vi "Initialization_K6221_ver1.0.vi"(4 "Input Comments String":string, 6 "output cluster":T1={"Main Sweep"=0, "Steps Config:"={"total points:"=0, "Step Delay (s)"=0.0, "Ini Delay (s)"=0.0, "# of steps:"=0}, "Temperature Control (ITC 503):"={"GPIB ADR"=0, "Change Heater?"={"Heater?"=FALSE, "Heater"=0}, "Change Temp?"={"Change T?"=FALSE, "Set T (K)"=0.0}, "Cluster"={"Heat Auto?"=FALSE, "Manual Heat?"=FALSE, "Heater (%)"=0.0}, "Change PID?"={"Change PID?"=FALSE, "P"=0.0, "I"=0.0, "D"=0.0}, "Change Para?"=FALSE, "Sensor"=1}, "Temperature Control (LS 340):"={"GPIB ADR"=0, "From (K)"=0.0, "To (K)"=0.0, "Rate (K/min)"=0.0, "Delta T (0.08K)"=0.0, "Temp. Header"="", "T Display Control"={"Ch B"=FALSE, "Ch C"=FALSE, "Ch D"=FALSE}}, "Magnet Control (IPS 120-10)"={"Action"=0, "Standby (s)"=0.0, "Heater on (s)"=0.0, "Sweep Setup "=[], "GPIB ADR"=0, "Change Para?"=FALSE}, "Keithley 6221 :"=[], "Measuring Instruments : "=[], "Lock-In SR7265 :"=[], "Deascription of \nthis measurement"="", "Instruments Config:"=[], "LS372 Bridge : 2"=[{"GPIB"=0, "Excitation"=0, "Autorange?"=FALSE, "Range"=0, "Current"=0, "Voltage"=0, "DataHeader"="Rx;Ry"}], "Magnet Control (CS4) 2"={"Action"=1, "Standby (s)"=0.0, "Heater on (s)"=300.0, "Sweep Setup "=[], "GPIB ADR"=0, "Change Para?"=FALSE}} {"Magnet Control (CS4) 2"."GPIB ADR" items=["None"=0, "25"=25]; "Magnet Control (CS4) 2"."Sweep Setup"."Rate in Range (T/min)" min=0.001 max=0.5 step=0.001; "Magnet Control (CS4) 2"."Sweep Setup"."Hold(min)" min=0.0; "Magnet Control (CS4) 2"."Sweep Setup"."Set Point (T)" min=-9.0 max=9.0 step=0.001; "Magnet Control (CS4) 2"."Action" items=["Up", "Down", "Pause", "Zero"]; "LS372 Bridge : 2"."Voltage" items=["2.00 uV"=1, "6.32 uV"=2, "20.0 uV"=3, "63.2 uV"=4, "200 uV"=5, "632 uV"=6, "2.0 mV"=7, "6.32 mV"=8]; "LS372 Bridge : 2"."Current" items=["1.00 pA"=1, "3.16 pA"=2, "10.0 pA"=3, "31.6 pA"=4, "100 pA"=5, "316 pA"=6, "1.00 nA"=7, "3.16 nA"=8, "10 nA"=9, "31.6 nA"=10, "100 nA"=11, "316 nA"=12, "1.00 uA"=13, "3.16 uA"=14, "10.0 uA"=15, "31.6 uA"=16, "100 uA"=17, "316 uA"=18, "1.00 mA"=19, "3.16 mA"=20, "10.0 mA"=21, "31.6 mA"=22]; "LS372 Bridge : 2"."Range" items=["2.0 m"=1, "6.32 m"=2, "20.0 m"=3, "63.2 m"=4, "200 m"=5, "632 m"=6, "2.00"=7, "6.32"=8, "20.0"=9, "63.2"=10, "200"=11, "632"=12, "2.00 k"=13, "6.32 k"=14, "20.0 k"=15, "63.2 k"=16, "200 k"=17, "632 k"=18, "2.00 M"=19, "6.32 M"=20, "20.0 M"=21, "63.2 M"=22]; "LS372 Bridge : 2"."Excitation" items=["Voltage", "Current"]; "LS372 Bridge : 2"."GPIB" items=["None"=0, "9"=9]; "Main Sweep" items=["Time", "DC Current", "Delta Current", "Pulse Delta Current", "Sine Current", "Lock-in Vosc"]; "Temperature Control (ITC 503):"."Sensor" items=["T2", "T3"]; "Magnet Control (IPS 120-10)"."Action" items=["Hold", "To Set point", "To Zero", "Clamp"]; "Keithley 6221 :"."Sweep Mode" items=["Linear", "Log", "Exp", "Inverse", "Manual"]}, 7 "error in (no error)":errorcluster, 10 "Input title array":string[](array[string])) -> (0 "error out":errorcluster, 1 "Output Comments string":string, 2 "output cluster 2":T1={"Main Sweep"=0, "Steps Config:"={"total points:"=0, "Step Delay (s)"=0.0, "Ini Delay (s)"=0.0, "# of steps:"=0}, "Temperature Control (ITC 503):"={"GPIB ADR"=0, "Change Heater?"={"Heater?"=FALSE, "Heater"=0}, "Change Temp?"={"Change T?"=FALSE, "Set T (K)"=0.0}, "Cluster"={"Heat Auto?"=FALSE, "Manual Heat?"=FALSE, "Heater (%)"=0.0}, "Change PID?"={"Change PID?"=FALSE, "P"=0.0, "I"=0.0, "D"=0.0}, "Change Para?"=FALSE, "Sensor"=1}, "Temperature Control (LS 340):"={"GPIB ADR"=0, "From (K)"=0.0, "To (K)"=0.0, "Rate (K/min)"=0.0, "Delta T (0.08K)"=0.0, "Temp. Header"="", "T Display Control"={"Ch B"=FALSE, "Ch C"=FALSE, "Ch D"=FALSE}}, "Magnet Control (IPS 120-10)"={"Action"=0, "Standby (s)"=0.0, "Heater on (s)"=0.0, "Sweep Setup "=[], "GPIB ADR"=0, "Change Para?"=FALSE}, "Keithley 6221 :"=[], "Measuring Instruments : "=[], "Lock-In SR7265 :"=[], "Deascription of \nthis measurement"="", "Instruments Config:"=[], "LS372 Bridge : 2"=[{"GPIB"=0, "Excitation"=0, "Autorange?"=FALSE, "Range"=0, "Current"=0, "Voltage"=0, "DataHeader"="Rx;Ry"}], "Magnet Control (CS4) 2"={"Action"=1, "Standby (s)"=0.0, "Heater on (s)"=300.0, "Sweep Setup "=[], "GPIB ADR"=0, "Change Para?"=FALSE}} {"Magnet Control (CS4) 2"."GPIB ADR" items=["None"=0, "25"=25]; "Magnet Control (CS4) 2"."Sweep Setup"."Rate in Range (T/min)" min=0.001 max=0.5 step=0.001; "Magnet Control (CS4) 2"."Sweep Setup"."Hold(min)" min=0.0; "Magnet Control (CS4) 2"."Sweep Setup"."Set Point (T)" min=-9.0 max=9.0 step=0.001; "Magnet Control (CS4) 2"."Action" items=["Up", "Down", "Pause", "Zero"]; "LS372 Bridge : 2"."Voltage" items=["2.00 uV"=1, "6.32 uV"=2, "20.0 uV"=3, "63.2 uV"=4, "200 uV"=5, "632 uV"=6, "2.0 mV"=7, "6.32 mV"=8]; "LS372 Bridge : 2"."Current" items=["1.00 pA"=1, "3.16 pA"=2, "10.0 pA"=3, "31.6 pA"=4, "100 pA"=5, "316 pA"=6, "1.00 nA"=7, "3.16 nA"=8, "10 nA"=9, "31.6 nA"=10, "100 nA"=11, "316 nA"=12, "1.00 uA"=13, "3.16 uA"=14, "10.0 uA"=15, "31.6 uA"=16, "100 uA"=17, "316 uA"=18, "1.00 mA"=19, "3.16 mA"=20, "10.0 mA"=21, "31.6 mA"=22]; "LS372 Bridge : 2"."Range" items=["2.0 m"=1, "6.32 m"=2, "20.0 m"=3, "63.2 m"=4, "200 m"=5, "632 m"=6, "2.00"=7, "6.32"=8, "20.0"=9, "63.2"=10, "200"=11, "632"=12, "2.00 k"=13, "6.32 k"=14, "20.0 k"=15, "63.2 k"=16, "200 k"=17, "632 k"=18, "2.00 M"=19, "6.32 M"=20, "20.0 M"=21, "63.2 M"=22]; "LS372 Bridge : 2"."Excitation" items=["Voltage", "Current"]; "LS372 Bridge : 2"."GPIB" items=["None"=0, "9"=9]; "Main Sweep" items=["Time", "DC Current", "Delta Current", "Pulse Delta Current", "Sine Current", "Lock-in Vosc"]; "Temperature Control (ITC 503):"."Sensor" items=["T2", "T3"]; "Magnet Control (IPS 120-10)"."Action" items=["Hold", "To Set point", "To Zero", "Clamp"]; "Keithley 6221 :"."Sweep Mode" items=["Linear", "Log", "Exp", "Inverse", "Manual"]}, 3 "Output title array":string[](array[string]), 8 "Output Mode Array":i32[](array[numeric]), 9 "VISA Refnum Out Array":refnum<visa-resource-name>[](array[refnum]))   [LabVIEW 2012]
doc: "Title Array: including time stamp, Temp (if selected), DCV, DCI, Vx, and Vy\nInstr GPIB ADR Array: If the instr is not selected, the GPIB ADR is equal to 0"
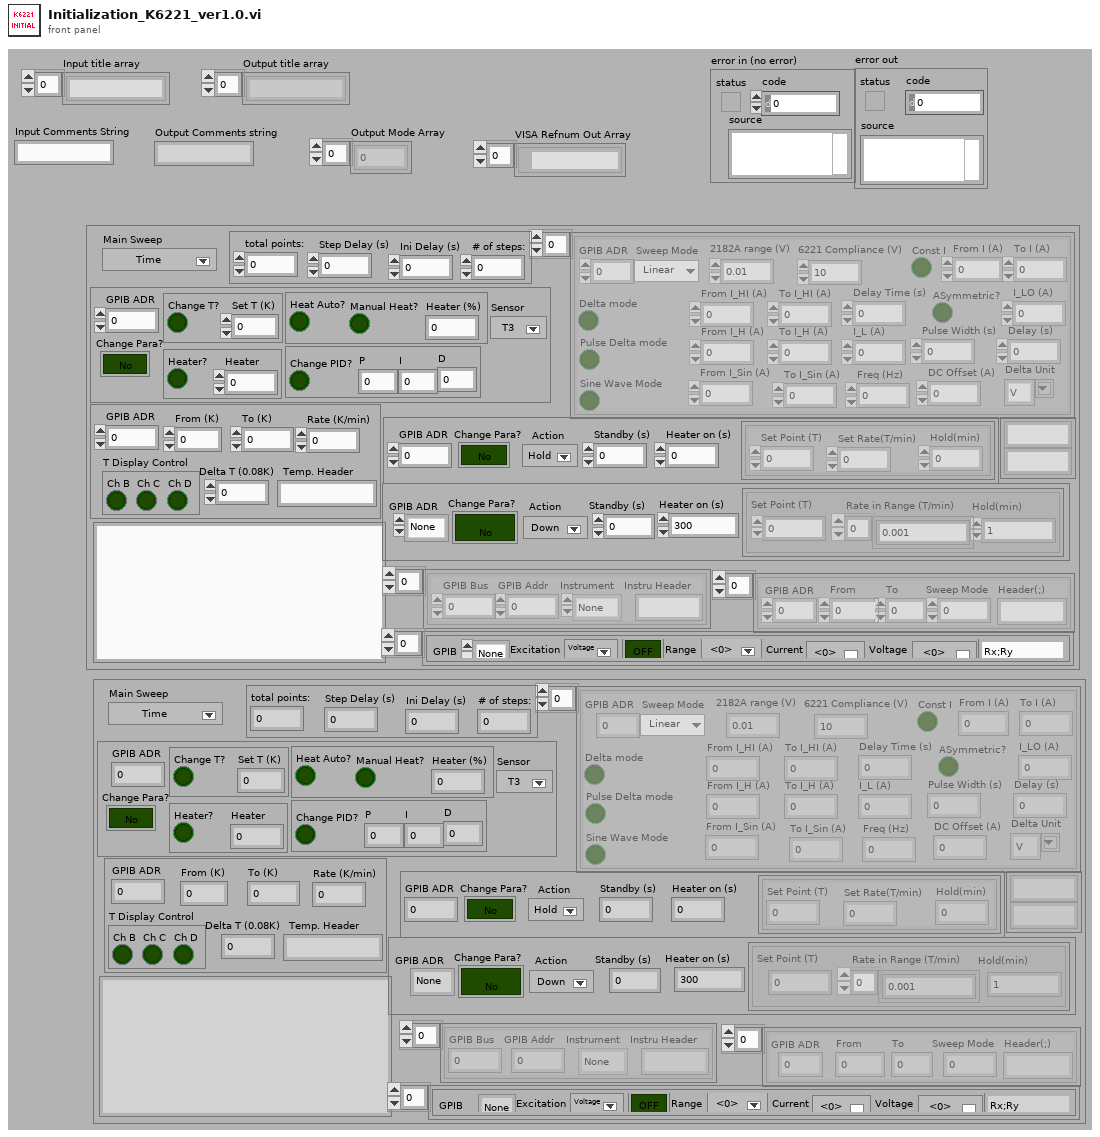
[diagram p1: front panel]
types:
  T1 = cluster{"Main Sweep":u8, "Steps Config:":cluster{"total points:":u32, "Step Delay (s)":dbl, "Ini Delay (s)":dbl, "# of steps:":u32}, "Temperature Control (ITC 503):":cluster{"GPIB ADR":u16, "Change Heater?":cluster{"Heater?":bool, "Heater":u8}, "Change Temp?":cluster{"Change T?":bool, "Set T (K)":dbl}, "Cluster":cluster{"Heat Auto?":bool, "Manual Heat?":bool, "Heater (%)":dbl}, "Change PID?":cluster{"Change PID?":bool, "P":dbl, "I":dbl, "D":dbl}, "Change Para?":bool, "Sensor":u16}, "Temperature Control (LS 340):":cluster{"GPIB ADR":u16, "From (K)":dbl, "To (K)":dbl, "Rate (K/min)":dbl, "Delta T (0.08K)":dbl, "Temp. Header":string, "T Display Control":cluster{"Ch B":bool, "Ch C":bool, "Ch D":bool}}, "Magnet Control (IPS 120-10)":cluster{"Action":u16, "Standby (s)":dbl, "Heater on (s)":dbl, "Sweep Setup ":cluster{"Set Point (T)":dbl, "Set Rate(T/min)":dbl, "Hold(min)":dbl}[], "GPIB ADR":u16, "Change Para?":bool}, "Keithley 6221 :":cluster{"Delta mode":bool, "Const I":bool, "Pulse Delta mode":bool, "Sine Wave Mode":bool, "From I_HI (A)":dbl, "From I (A)":dbl, "I_LO (A)":dbl, "From I_H (A)":dbl, "I_L (A)":dbl, "Freq (Hz)":dbl, "From I_Sin (A)":dbl, "DC Offset (A)":dbl, "Delay Time (s)":dbl, "Pulse Width (s)":dbl, "Delay (s)":dbl, "To I (A)":dbl, "ASymmetric?":bool, "To I_HI (A)":dbl, "To I_H (A)":dbl, "To I_Sin (A)":dbl, "GPIB ADR":u16, "Sweep Mode":u8, "Delta Unit":string, "2182A range (V)":dbl, "6221 Compliance (V)":dbl}[], "Measuring Instruments : ":cluster{"GPIB Bus":dbl, "GPIB Addr":dbl, "Instrument":enum16{"None", "HP34401DMM", "Lockin 7265", "HP3456/7A", "HP3478A", "HP3325FG", "Keithley2182A"}, "Instru Header":string}[], "Lock-In SR7265 :":cluster{"GPIB ADR":u16, "From":dbl, "To":dbl, "Header(;)":string, "Sweep Mode":u8}[], "Deascription of \nthis measurement":string, "Instruments Config:":string[][], "LS372 Bridge : 2":cluster{"GPIB":u16, "Excitation":u16, "Autorange?":bool, "Range":u16, "Current":u16, "Voltage":u16, "DataHeader":string}[], "Magnet Control (CS4) 2":cluster{"Action":u16, "Standby (s)":dbl, "Heater on (s)":dbl, "Sweep Setup ":cluster{"Set Point (T)":dbl, "Hold(min)":dbl, "Rate in Range (T/min)":dbl[]}[], "GPIB ADR":u16, "Change Para?":bool}}
  T2 = cluster{"Delta mode":bool, "Const I":bool, "Pulse Delta mode":bool, "Sine Wave Mode":bool, "From I_HI (A)":dbl, "From I (A)":dbl, "I_LO (A)":dbl, "From I_H (A)":dbl, "I_L (A)":dbl, "Freq (Hz)":dbl, "From I_Sin (A)":dbl, "DC Offset (A)":dbl, "Delay Time (s)":dbl, "Pulse Width (s)":dbl, "Delay (s)":dbl, "To I (A)":dbl, "ASymmetric?":bool, "To I_HI (A)":dbl, "To I_H (A)":dbl, "To I_Sin (A)":dbl, "GPIB ADR":u16, "Sweep Mode":u8, "Delta Unit":string, "2182A range (V)":dbl, "6221 Compliance (V)":dbl}[]
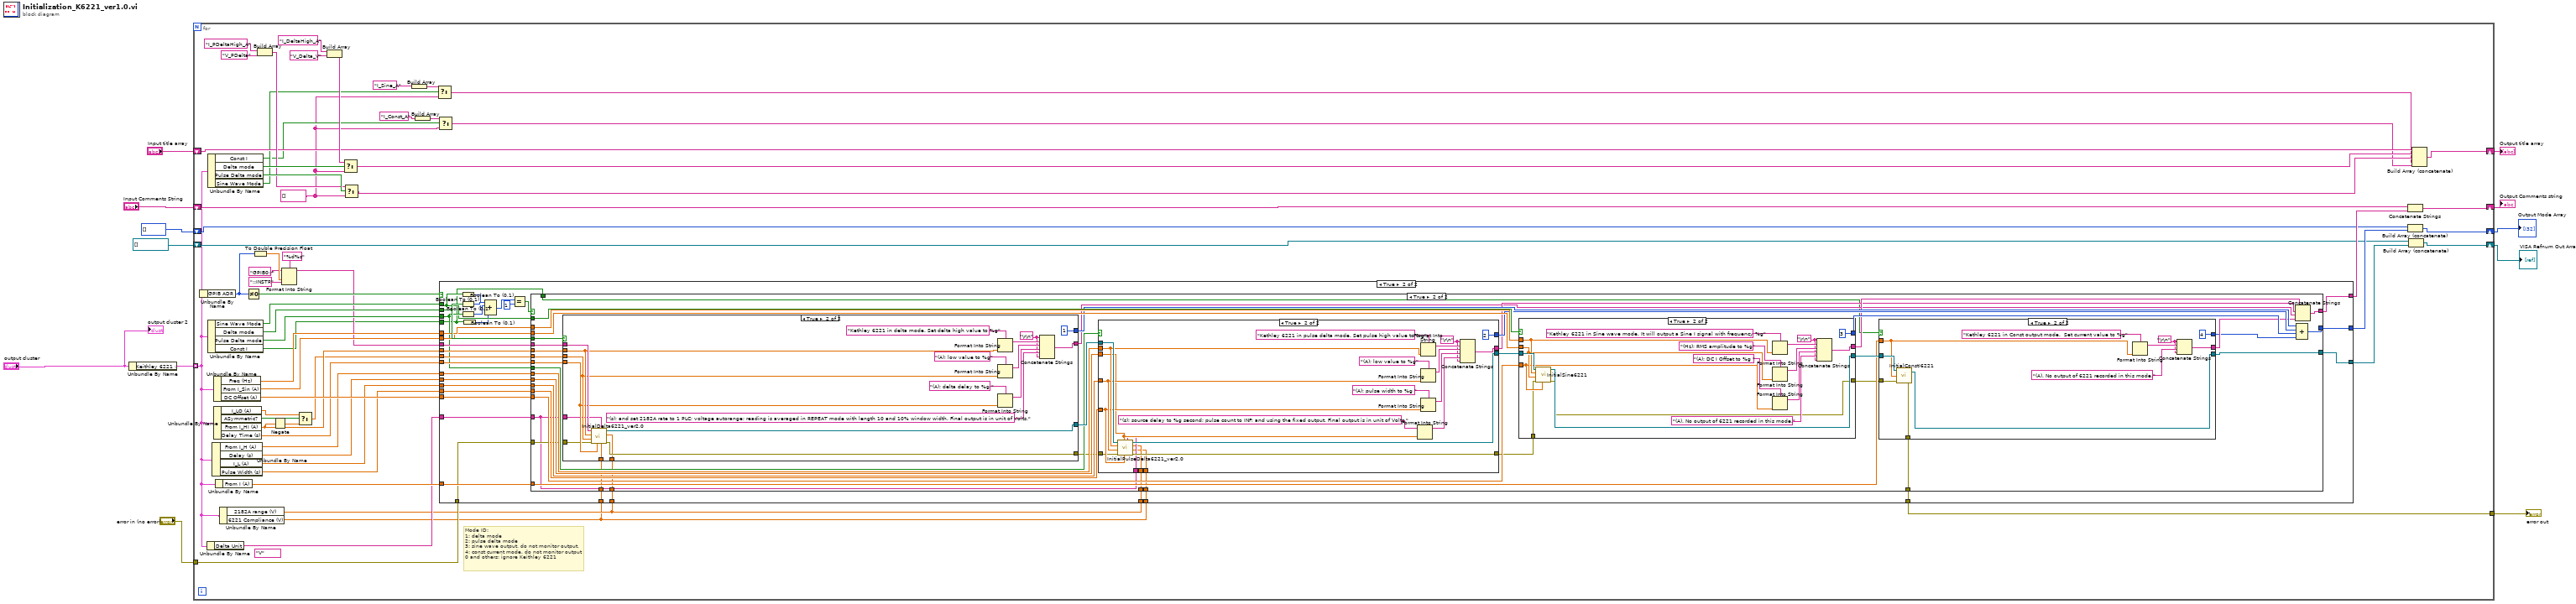
[diagram p0: block diagram]
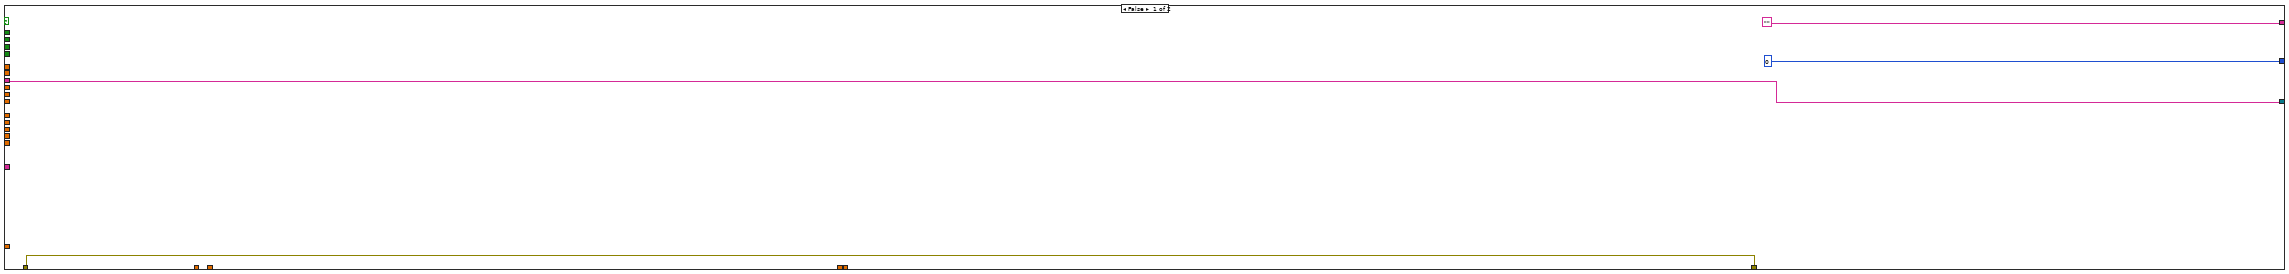
[diagram p2: hidden frame]
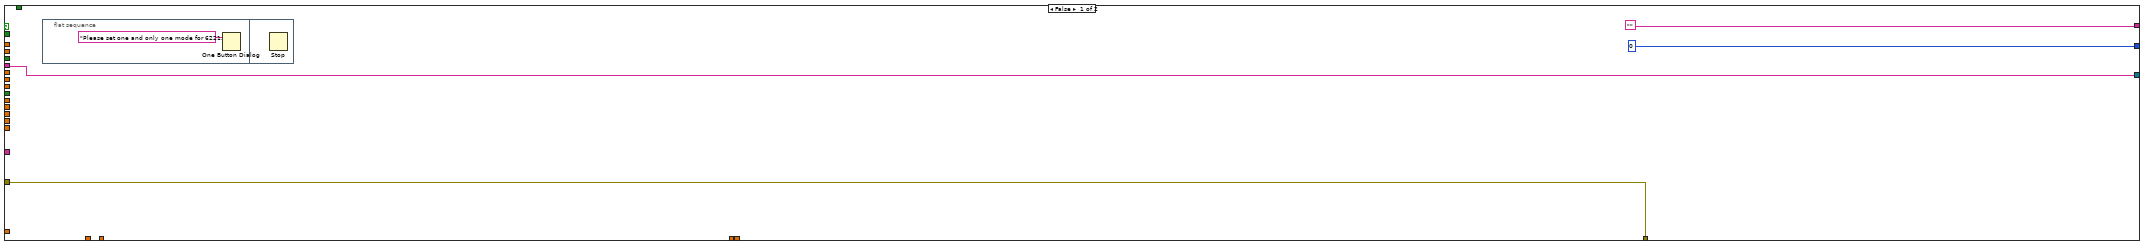
[diagram p3: hidden frame]
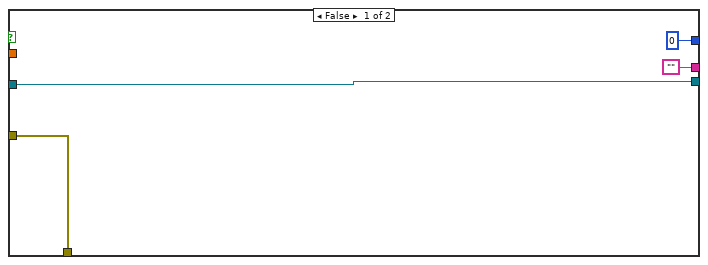
[diagram p4: hidden frame]
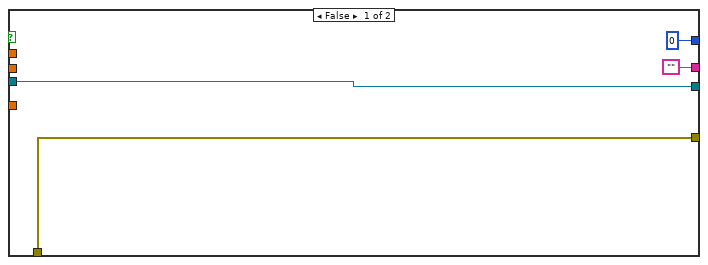
[diagram p5: hidden frame]
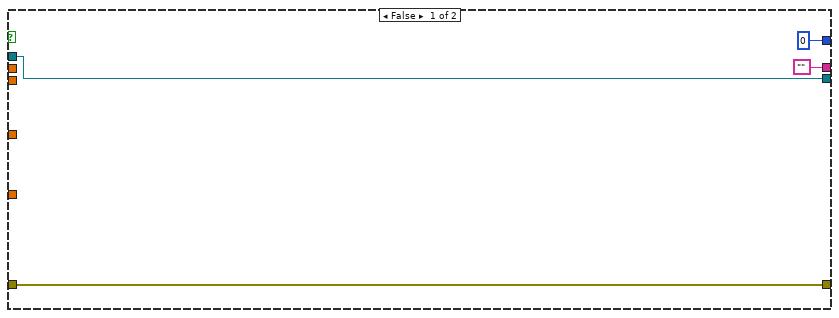
[diagram p6: hidden frame]
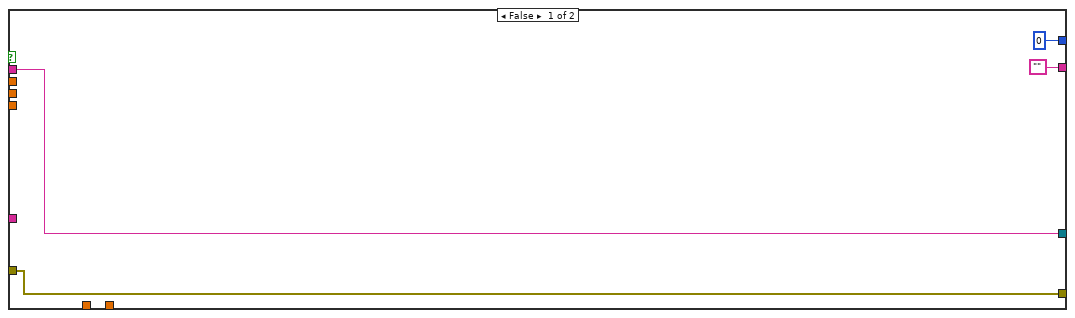
[diagram p7: hidden frame]
diagram:
  n1 = Unbundle By Name("output cluster") -> ("Keithley 6221 :"=w12:T2)
  n2 = for {
    tunnel: w12 -> [w15] mode=indexing
    tunnel: "error in (no error)" -> [w41]
    shift-right: [w37] -> w5
    shift-left: "Input Comments String" -> [w46]
    shift-right: [w43] -> w8
    shift-left: i32[] [] ("appended array") -> [w45]
    shift-right: [w42] -> w7
    shift-left: refnum<visa-resource-name>[] [] ("appended array") -> [w44]
    tunnel: [w40] -> w6
    shift-right: [w28] -> w2
    shift-left: "Input title array" -> [w29]
    (unwired) "V" ("Unit")
    w21 = string[] [] ("appended array")
    # "Mode ID:\n1: delta mode\n2: pulse delta mode\n3: sine wave output. do not monitor output.\n4: const current mode. do not monitor output\n0 and others: ignore Keithley 6221"
    n3 = Unbundle By Name(w15) -> ("GPIB ADR"=w69:u16)
    n4 = Unbundle By Name(w15) -> ("Delta Unit"=w16:string)
    n5 = Unbundle By Name(w15) -> ("Const I"=w22:bool, "Delta mode"=w39:bool, "Pulse Delta mode"=w38:bool, "Sine Wave Mode"=w27:bool)
    n6 = Unbundle By Name(w15) -> ("Sine Wave Mode"=w67:bool, "Delta mode"=w66:bool, "Pulse Delta mode"=w65:bool, "Const I"=w51:bool)
    n7 = Unbundle By Name(w15) -> ("From I_H (A)"=w55:dbl, "Delay (s)"=w54:dbl, "I_L (A)"=w53:dbl, "Pulse Width (s)"=w52:dbl)
    n8 = Unbundle By Name(w15) -> ("Freq (Hz)"=w64:dbl, "From I_Sin (A)"=w63:dbl, "DC Offset (A)"=w62:dbl)
    n9 = Unbundle By Name(w15) -> ("I_LO (A)"=w59:dbl, "ASymmetric?"=w60:bool, "From I_HI (A)"=w58:dbl, "Delay Time (s)"=w56:dbl)
    n10 = Unbundle By Name(w15) -> ("From I (A)"=w50:dbl)
    n11 = Unbundle By Name(w15) -> ("2182A range (V)"=w14:dbl, "6221 Compliance (V)"=w13:dbl)
    n12 = Not Equal To 0?(x=w69) -> (x != 0?=w68:bool)
    n13 = To Double Precision Float(number=w69) -> (double precision float=w72:dbl)
    n14 = Build Array("I_PDeltaHigh_A" ("Removes all labels from the string"), "V_PDelta" ("Removes all labels from the string")) -> (w31:string[])
    n15 = Negate(x=w58) -> (-x=w23:dbl)
    n16 = Format Into String(format string="%d%s" ("Removes all labels from the string"), initial string="GPIB0::", w72, "::INSTR") -> (resulting string=w61:string)  [unwired: 1 in, 1 out]
    n17 = Select(t=w59, s=w60, f=w23) -> (s? t:f=w57:dbl)
    n18 = Build Array("I_DeltaHigh_A" ("Removes all labels from the string"), "V_Delta_V" ("Removes all labels from the string")) -> (w34:string[])
    n19 = Select(t=w34, s=w39, f=w21) -> (s? t:f=w30:string[])
    n20 = Select(t=w31, s=w38, f=w21) -> (s? t:f=w24:string[])
    n21 = Build Array("I_Sine_A" ("Removes all labels from the string")) -> (w25:string[])
    n22 = Build Array("I_Const_A" ("Removes all labels from the string")) -> (w20:string[])
    n23 = Select(t=w25, s=w27, f=w21) -> (s? t:f=w18:string[])
    n24 = Select(t=w20, s=w22, f=w21) -> (s? t:f=w17:string[])
    n25 = case shown="True" w68 {
      tunnel: w66 -> [_ w103]
      tunnel: w65 -> [_ w92]
      tunnel: w67 -> [_ w91]
      tunnel: w61 -> [w77 w104]
      tunnel: w58 -> [_ w102]
      tunnel: w57 -> [_ w101]
      tunnel: w56 -> [_ w100]
      tunnel: [w77 w99] -> w47
      tunnel: w55 -> [_ w98]
      tunnel: w53 -> [_ w97]
      tunnel: w52 -> [_ w96]
      tunnel: w64 -> [_ w95]
      tunnel: w63 -> [_ w94]
      tunnel: w62 -> [_ w93]
      tunnel: [0 w90] -> w48
      tunnel: ["" w85] -> w49
      tunnel: w54 -> [_ w89]
      tunnel: w51 -> [_ w87]
      tunnel: w50 -> [_ w86]
      tunnel: w41 -> [w74 w84]
      tunnel: [w74 w83] -> w40
      tunnel: w16 -> [_ w82]
      tunnel: w14 -> [_ w81]
      tunnel: w13 -> [_ w80]
      tunnel: w14 -> [_ w79]
      tunnel: w13 -> [_ w78]
      frame False {
      }
      frame True {
        n26 = Boolean To (0,1)(Boolean=w91) -> (0, 1=w108:i16)
        n27 = Boolean To (0,1)(Boolean=w103) -> (0, 1=w110:i16)
        n28 = Boolean To (0,1)(Boolean=w92) -> (0, 1=w109:i16)
        n29 = Boolean To (0,1)(Boolean=w87) -> (0, 1=w88:i16)
        n30 = Compound Arithmetic op=ADD(w110, w109, w108, w88) -> (w107:i16)
        n31 = Equal?(x=w107, y=i16 1) -> (x = y?=w105:bool)
        n32 = case shown="True" w105 {
          tunnel: w104 -> [w114 w154]
          tunnel: w103 -> [_ w155]
          tunnel: w102 -> [_ w153]
          tunnel: w101 -> [_ w152]
          tunnel: w100 -> [_ w151]
          tunnel: [w114 w126] -> w99
          tunnel: w98 -> [_ w149]
          tunnel: w97 -> [_ w148]
          tunnel: w96 -> [_ w147]
          tunnel: w95 -> [_ w146]
          tunnel: w94 -> [_ w145]
          tunnel: w93 -> [_ w144]
          tunnel: w92 -> [_ w143]
          tunnel: w91 -> [_ w142]
          tunnel: [0 w140] -> w90
          tunnel: ["" w133] -> w85
          tunnel: w89 -> [_ w132]
          tunnel: w87 -> [_ w130]
          tunnel: w86 -> [_ w129]
          tunnel: w84 -> [w111 w125]
          tunnel: [w111 w121] -> w83
          tunnel: w82 -> [_ w120]
          tunnel: w81 -> [_ w119]
          tunnel: w80 -> [_ w118]
          tunnel: w79 -> [_ w117]
          tunnel: w78 -> [_ w116]
          frame False {
            n33 = flat-sequence {
              frame #0 {
                n34 = One Button Dialog(message="Please set one and only one mode for 6221.") -> ()  [unwired: 1 in, 1 out]
              }
              frame #1 {
                n35 = Stop() -> ()  [unwired: 1 in]
              }
            }
          }
          frame True {
            n36 = case shown="True" w155 {
              tunnel: w154 -> [w221 w241]
              tunnel: w153 -> [_ w232]
              tunnel: w152 -> [_ w230]
              tunnel: w151 -> [_ w229]
              tunnel: [w221 w240] -> w150
              tunnel: [0 1] -> w139
              tunnel: ["" w228] -> w134
              tunnel: w125 -> [w218 w226]
              tunnel: [w218 w225] -> w124
              tunnel: w120 -> [_ w224]
              tunnel: w119 -> [_ w223]
              tunnel: w118 -> [_ w222]
              frame False {
              }
              frame True {
                w227 = "\r\n"
                n37 = call "InitialDelta6221_ver2.0.vi"("NV2182A range (V)"=w223, "Keithley6221 Compliance (V)"=w222, "Unit"=w224, "Delay In (s)"=w229, "error in (no error)"=w226, "Low Level In (A)"=w230, "High Level In (A)"=w232, "VISA Refnum in"=w241) -> ("error out"=w225:errorcluster, "VISA Refnum out"=w240:refnum<visa-resource-name>)  [unwired: 2 in]
                n38 = Format Into String(format string="Kethley 6221 in delta mode. Set delta high value to %g", w232) -> (resulting string=w237:string)  [unwired: 2 in, 1 out]
                n39 = Format Into String(format string="(A); low value to %g", w230) -> (resulting string=w236:string)  [unwired: 2 in, 1 out]
                n40 = Format Into String(format string="(A); delta delay to %g ", w229) -> (resulting string=w234:string)  [unwired: 2 in, 1 out]
                n41 = Concatenate Strings(w227, w237, w236, w234, "(s); and set 2182A rate to 1 PLC; voltage autorange; reading is averaged in REPEAT mode with length 10 and 10% window width. Final output is in unit of Volts.", w227) -> (w228:string)
              }
            }
            n42 = case shown="True" w143 {
              tunnel: w149 -> [_ w214]
              tunnel: w148 -> [_ w211]
              tunnel: w147 -> [_ w208]
              tunnel: w150 -> [w195 w217]
              tunnel: [w195 w216] -> w141
              tunnel: [0 2] -> w138
              tunnel: ["" w205] -> w135
              tunnel: w132 -> [_ w202]
              tunnel: w124 -> [w192 w200]
              tunnel: [w192 w199] -> w122
              tunnel: w120 -> [_ w198]
              tunnel: w117 -> [_ w197]
              tunnel: w116 -> [_ w196]
              frame False {
              }
              frame True {
                w201 = "\r\n"
                n43 = call "InitialPulseDelta6221_ver2.0.vi"("Keithley6221 Compliance (V)"=w196, "NV2182A range (V)"=w197, "Unit"=w198, "Pluse Width  In (s)"=w208, "Delay Time (s)"=w202, "error in (no error)"=w200, "Low Level In (A)"=w211, "High Level In (A)"=w214, "VISA Refnum in"=w217) -> ("error out"=w199:errorcluster, "VISA Refnum out"=w216:refnum<visa-resource-name>)  [unwired: 1 in]
                n44 = Format Into String(initial string="(s); source delay to %g second; pulse count to INF; and using the fixed output. Final output is in unit of Volts.", w202) -> (resulting string=w203:string)  [unwired: 2 in, 1 out]
                n45 = Format Into String(format string="Kethley 6221 in pulse delta mode. Set pulse high value to %g", w214) -> (resulting string=w210:string)  [unwired: 2 in, 1 out]
                n46 = Format Into String(format string="(A); low value to %g", w211) -> (resulting string=w209:string)  [unwired: 2 in, 1 out]
                n47 = Format Into String(format string="(A); pulse width to %g ", w208) -> (resulting string=w206:string)  [unwired: 2 in, 1 out]
                n48 = Concatenate Strings(w201, w210, w209, w206, w203, w201) -> (w205:string)
              }
            }
            n49 = case shown="True" w142 {
              tunnel: w141 -> [w174 w191]
              tunnel: w146 -> [_ w180]
              tunnel: w145 -> [_ w179]
              tunnel: w144 -> [_ w178]
              tunnel: [w174 w190] -> w131
              tunnel: [0 3] -> w137
              tunnel: ["" w181] -> w136
              tunnel: [w171 w176] -> w123
              tunnel: w122 -> [w171 w175]
              frame False {
              }
              frame True {
                w177 = "\r\n"
                n50 = call "InitialSine6221.vi"("DC Offset In (A)"=w178, "error in (no error)"=w175, "Amplitude In (A)"=w179, "Frequency In (Hz)"=w180, "VISA Refnum in"=w191) -> ("error out"=w176:errorcluster, "VISA Refnum out"=w190:refnum<visa-resource-name>)  [unwired: 5 in]
                n51 = Format Into String(format string="Kethley 6221 in Sine wave mode. It will output a Sine I signal with frequency %g", w180) -> (resulting string=w186:string)  [unwired: 2 in, 1 out]
                n52 = Format Into String(format string="(Hz); RMS amplitude to %g", w179) -> (resulting string=w185:string)  [unwired: 2 in, 1 out]
                n53 = Format Into String(format string="(A); DC I Offset to %g ", w178) -> (resulting string=w183:string)  [unwired: 2 in, 1 out]
                n54 = Concatenate Strings(w177, w186, w185, w183, "(A). No output of 6221 recorded in this mode.", w177) -> (w181:string)
              }
            }
            n55 = case shown="True" w130 {
              tunnel: w131 -> [w159 w170]
              tunnel: w129 -> [_ w162]
              tunnel: [w159 w169] -> w126
              tunnel: [0 4] -> w127
              tunnel: ["" w164] -> w128
              tunnel: w123 -> [w156 w161]
              tunnel: [w156 w160] -> w121
              frame False {
              }
              frame True {
                w163 = "\r\n"
                n56 = call "InitialConstI6221.vi"("error in (no error)"=w161, "Amplitude In (A)"=w162, "VISA Refnum in"=w170) -> ("error out"=w160:errorcluster, "VISA Refnum out"=w169:refnum<visa-resource-name>)
                n57 = Format Into String(format string="Kethley 6221 in Const output mode.  Set current value to %g", w162) -> (resulting string=w166:string)  [unwired: 2 in, 1 out]
                n58 = Concatenate Strings(w163, w166, "(A). No output of 6221 recorded in this mode.", w163) -> (w164:string)
              }
            }
            n59 = Concatenate Strings(w136, w135, w134, w128) -> (w133:string)
            n60 = Compound Arithmetic op=ADD(w139, w138, w137, w127) -> (w140:i32)
          }
        }
      }
    }
    n61 = Concatenate Strings(w46, w49) -> (w37:string)
    n62 = Build Array (concatenate)(w45, w48) -> (w43:i32[])
    n63 = Build Array (concatenate)(w44, w47) -> (w42:refnum<visa-resource-name>[])
    n64 = Build Array (concatenate)(w29, w30, w24, w18, w17) -> (w28:string[])
  }
  "error out" <- w6
  "Output Mode Array" <- w8
  "VISA Refnum Out Array" <- w7
  "Output Comments string" <- w5
  "Output title array" <- w2
  "output cluster 2" <- "output cluster"
